vi "SMBus Get Alert.vi"(9 "SMBUSIndex":i32, 10 "DevIndex":i32, 11 "DevType":i32) -> (2 "function return":i32, 3 "pAlertFlag":u8)   [LabVIEW 2010, in "ControlSMBus.lvlib"]
doc: "int WINAPI SMBus_GetAlert(int DevType,int DevIndex,int SMBUSIndex,unsigned char *pAlertFlag);"
uses:
  ControlSMBus.lvlib
  ControlSMBus/Ginkgo_Driver.dll
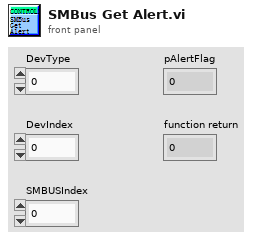
[diagram p1: front panel]
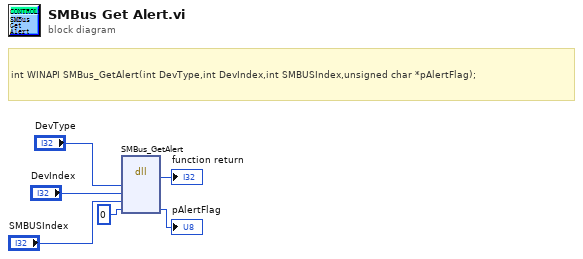
[diagram p0: block diagram]
diagram:
  # "int WINAPI SMBus_GetAlert(int DevType,int DevIndex,int SMBUSIndex,unsigned char *pAlertFlag);"
  n1 = dll-call lib="E:/Project/vt_ginkgo/truck/Ginkgo Driver/vs2010/Ginkgo_USB-I2C&SPI&CAN_API_v2.0.3.3/lib/labview_32bit/ControlSMBus/Ginkgo_Driver.*" fn="SMBus_GetAlert"("DevType"="DevType", "DevIndex"="DevIndex", "SMBUSIndex"="SMBUSIndex", "pAlertFlag"=u8 0) -> (→"function return":i32, "pAlertFlag"=→"pAlertFlag":u8)  [unwired: 6 in, 2 out]
